vi "benchmark-jitter.vi"(10 "wait (s)":dbl=0.001, 11 "iterations":i32=1000) -> (0 "mean (s)":dbl format="%#_6f", 1 "max value":dbl format="%#_6f", 2 "min value (s)":dbl format="%#_6f", 3 "data":dbl[][](array[numeric]), 4 "lag (s)":dbl, 6 "duration (s)":dbl)   [LabVIEW 2020]
uses:
  60dc524a-c1be-3fe3-a074-7e4ffbe5cd3f.vi
  <vilib>/Analysis/baseanly.llb/Mean (DBL).vi
  <vilib>/Analysis/NI_AALBase.lvlib
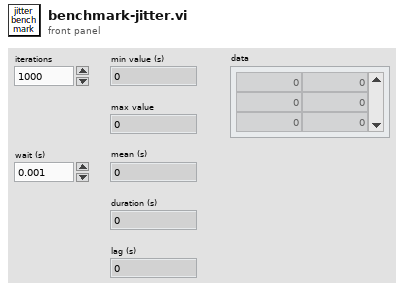
[diagram p1: front panel]
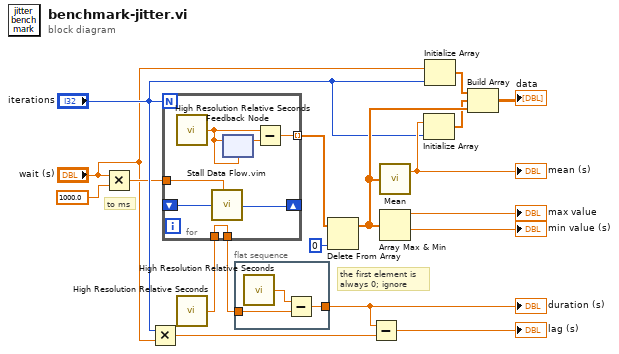
[diagram p0: block diagram]
diagram:
  # "to ms"
  # "the first element is \nalways 0; ignore"
  n1 = Multiply(x="wait (s)", y=1000.0) -> (x*y=w2:dbl)
  n2 = Multiply(x="iterations", y="wait (s)") -> (x*y=w4:dbl)
  n3 = call <vilib>:"High Resolution Relative Seconds.vi"() -> ("relative seconds"=w10:dbl)
  n4 = for {
    N: "iterations" -> [_]
    tunnel: [w24] -> w16 mode=indexing
    shift-right: [w20] -> _
    shift-left: _ -> [w22]
    tunnel: w2 -> [w21]
    tunnel: w10 -> [w19]
    tunnel: [w19] -> w9
    n5 = call <vilib>:"High Resolution Relative Seconds.vi"() -> ("relative seconds"=w23:dbl)
    n6 = call "Stall Data Flow.vim"("value in"=w22, "milliseconds to wait"=w21) -> ("value out"=w20:u32)  [unwired: 1 out]
    n7 = feedback-in #1(w23) -> ()
    n8 = feedback #1(w23) -> (w25:dbl)
    n9 = Subtract(x=w23, y=w25) -> (x-y=w24:dbl)
  }
  n10 = flat-sequence {
    tunnel: w9 -> [w27]
    tunnel: [w26] -> w7
    frame #0 {
      n11 = call <vilib>:"High Resolution Relative Seconds.vi"() -> ("relative seconds"=w28:dbl)
      n12 = Subtract(x=w28, y=w27) -> (x-y=w26:dbl)
    }
  }
  n13 = Delete From Array(array=w16, index=0) -> (array with subset deleted=w12:dbl[])  [unwired: 1 in, 1 out]
  n14 = Subtract(x=w7, y=w4) -> (x-y=→"lag (s)":dbl)
  n15 = call-poly <vilib>:"Mean.vi"("X"=w12) -> ("mean"=w14:dbl)  [unwired: 1 out]
  "mean (s)" <- w14
  n16 = Array Max & Min(array=w12) -> (max value=→"max value":dbl, min value=→"min value (s)":dbl)  [unwired: 2 out]
  n17 = Initialize Array(w14, "iterations") -> (w11:dbl[])
  n18 = Initialize Array("wait (s)", "iterations") -> (w13:dbl[])
  n19 = Build Array(w13, w11, w12) -> (→"data":dbl[][])
  "duration (s)" <- w7
